vi "Init Data BDD.vi"(8 "errin":errorcluster, 10 "Type":string, 11 "SN":string) -> (0 "error out":errorcluster, 3 "chaîne concaténée":string)   [LabVIEW 2020]
doc: "On créer le produit dans la base"
uses:
  VarGLO/Global var.vi
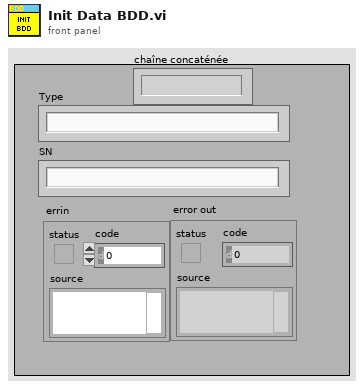
[diagram p1: front panel]
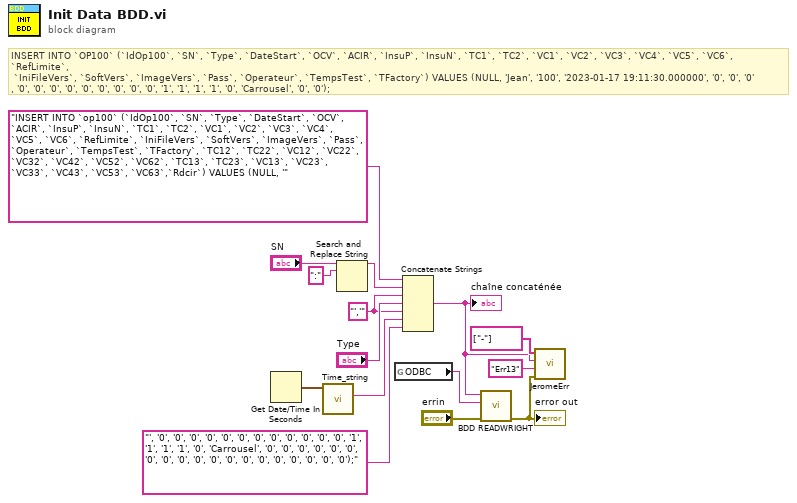
[diagram p0: block diagram]
diagram:
  w8 = "','" ("chaîne")
  # "INSERT INTO `OP100` (`IdOp100`, `SN`, `Type`, `DateStart`, `OCV`, `ACIR`, `InsuP`, `InsuN`, `TC1`, `TC2`, `VC1`, `VC2`, `VC3`, `VC4`, `VC5`, `VC6`, `RefLimite`,\n `IniFileVers`, `SoftVers`, `ImageVers`, `Pass`, `Operateur`, `TempsTest`, `TFactory`) VALUES (NULL, 'Jean', '100', '2023-01-17 19:11:30.000000', '0', '0', '0'\n, '0', '0', '0', '0', '0', '0', '0', '0', '0', '1', '1', '1', '1', '0', 'Carrousel', '0', '0');"
  n1 = Get Date/Time In Seconds() -> (seconds since 1Jan1904=w10:timestamp)
  n2 = call <userlib>:"Time_string.vi"("h in"=w10) -> ("heure sql"=w9:string)  [unwired: 9 in, 1 out]
  n3 = Search and Replace String ("Rechercher et remplacer une chaîne")(input string="SN", search string=":" ("chaîne recherchée")) -> (result string=w12:string)  [unwired: 6 in, 3 out]
  n4 = global read "Global var.vi" "ODBC"() -> (w1:string)
  n5 = Concatenate Strings("INSERT INTO `op100` (`IdOp100`, `SN`, `Type`, `DateStart`, `OCV`, `ACIR`, `InsuP`, `InsuN`, `TC1`, `TC2`, `VC1`, `VC2`, `VC3`, `VC4`, `VC5`, `VC6`, `RefLimite`, `IniFileVers`, `SoftVers`, `ImageVers`, `Pass`, `Operateur`, `TempsTest`, `TFactory`, `TC12`, `TC22`, `VC12`, `VC22`, `VC32`, `VC42`, `VC52`, `VC62`, `TC13`, `TC23`, `VC13`, `VC23`, `VC33`, `VC43`, `VC53`, `VC63`,`Rdcir`) VALUES (NULL, '" ("chaîne"), w12, w8, "Type", w8, w9, "', '0', '0', '0', '0', '0', '0', '0', '0', '0', '0', '0', '0', '1', '1', '1', '1', '0', 'Carrousel', '0', '0', '0', '0', '0', '0', '0', '0', '0', '0', '0', '0', '0', '0', '0', '0', '0', '0', '0');" ("chaîne")) -> (w2:string)
  "chaîne concaténée" <- w2
  n6 = call <userlib>:"BDD READWRIGHT.vi"("errin"="errin", "DSN name"=w1, "Instruction"=w2) -> ("error out"=w3:errorcluster)  [unwired: 7 in, 1 out]
  "error out" <- w3
  n7 = call "JeromeErr.vi"("Errin"=w3, "CodeERR"="Err13", "RequetteSQL"=w2, "RetourSQL"=string[] ["-"]) -> ()  [unwired: 8 in]
